vi "SpectrumViewer.vi"() -> ()   [LabVIEW 2016]
uses:
  <vilib>/Utility/miscctls.llb/LVPointDoubleTypeDef.ctl
  <vilib>/GPower/Numeric/Library/Average/AvrgDBL.vi
  <vilib>/Analysis/baseanly.llb/Mean (DBL).vi
  <vilib>/Utility/file.llb/Write Delimited Spreadsheet (DBL).vi
  <vilib>/Analysis/NI_AALBase.lvlib
  <vilib>/GPower/Numeric/GPNumeric.lvlib
panel:
  in  "Wavelength maximum":i32(slide)=374 min=374 max=761 step=1 scale=374.0..761.0
  in  "File Path":path
  in  "Save":bool
  out "Spectrum at cursor":i16[](graph)
  in  "Wavelength minimum":i32(slide)=374 min=374 max=761 step=1 scale=374.0..761.0
  in  "Intensity Graph":sgl[][](graph)
  in  "Quit":bool
  out "error out":errorcluster
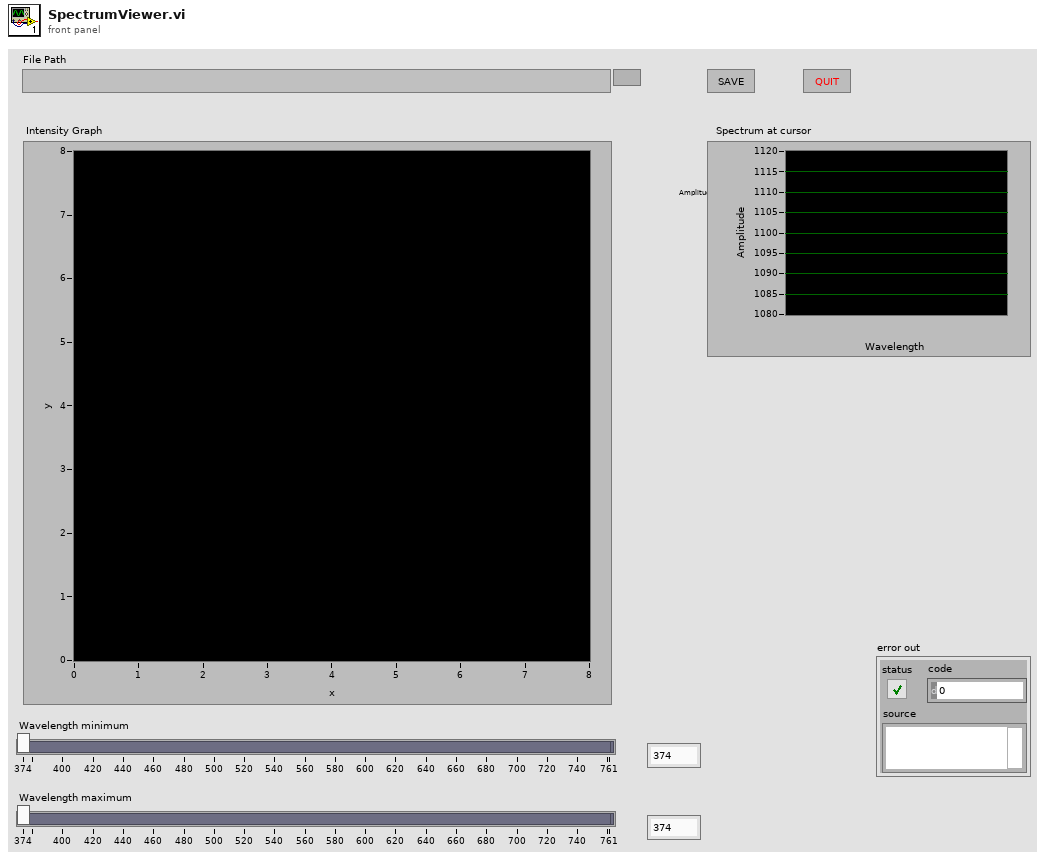
[diagram p1: front panel]
types:
  T1 = typedef "LVPointDoubleTypeDef.ctl" = cluster{"X":dbl, "Y":dbl}
  T2 = typedef "Image Type" = u32
  T3 = typedef "IMAQ Image.ctl" = refnum<image>
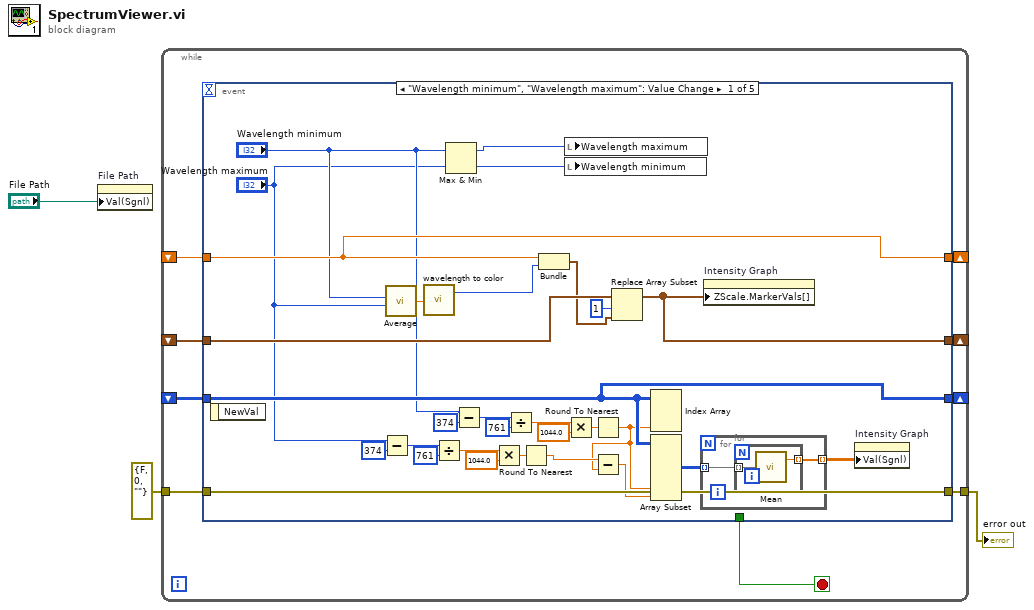
[diagram p0: block diagram]
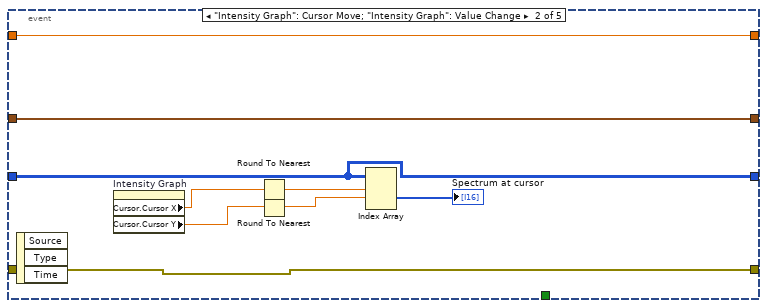
[diagram p2: hidden frame]
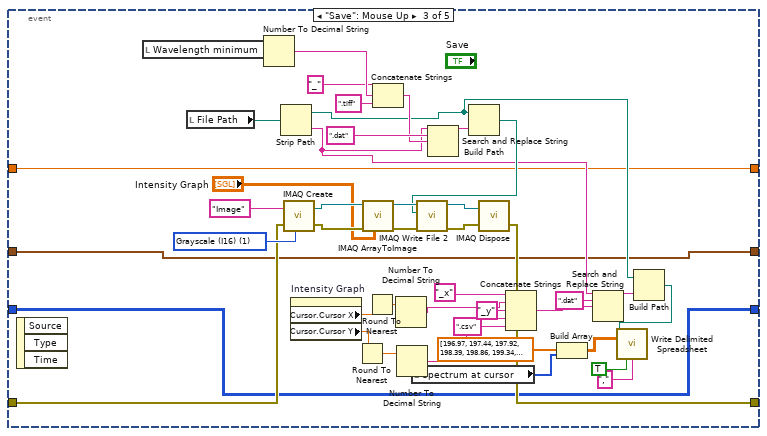
[diagram p3: hidden frame]
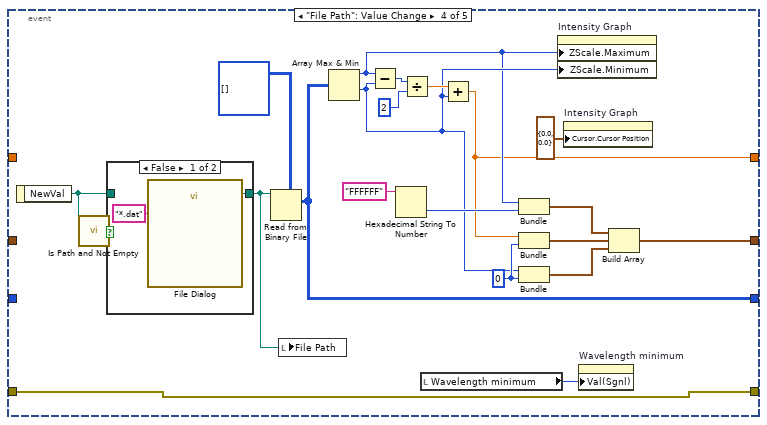
[diagram p4: hidden frame]
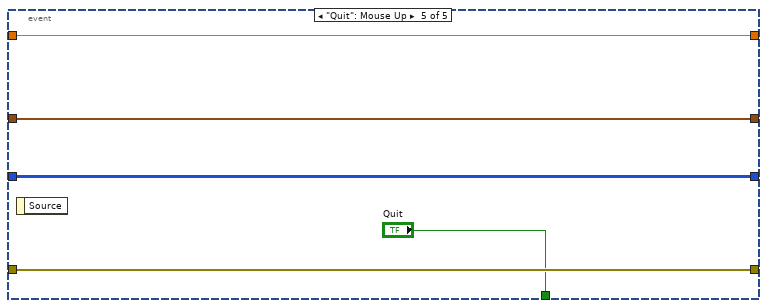
[diagram p6: hidden frame]
diagram:
  n1 = property on="File Path" class="Path"("Val(Sgnl)"="File Path") -> ()  [unwired: 2 in, 2 out]
  n2 = while {
    tunnel: errorcluster {"status"=FALSE, "code"=0, "source"=""} ("error out") -> [w11]
    tunnel: [w10] -> w3
    shift-right: [w6] -> _
    shift-left: _ -> [w12]
    shift-right: [w5] -> _
    shift-left: _ -> [w8]
    shift-right: [w4] -> _
    shift-left: _ -> [w7]
    stop <- w9 stop-if-true
    n3 = event shown="[0] \"Wavelength minimum\", \"Wavelength maximum\": Value Change" {
      selector: _ -> [_ _ _ _ _]
      dyn-events: _ -> [_ _ _ _ _]
      timeout: _ -> [_ _ _ _ _]
      tunnel: w12 -> [w23 w51 w64 _ w126]
      tunnel: w11 -> [w42 w52 w89 w112 w127]
      tunnel: [w42 w52 w90 w112 w127] -> w10
      tunnel: [_ _ _ _ "Quit"] -> w9
      tunnel: w8 -> [w41 w50 w58 _ w125]
      tunnel: w7 -> [w30 w49 w57 _ w124]
      tunnel: [w23 w51 w64 w116 w126] -> w6
      tunnel: [w31 w50 w58 w108 w125] -> w5
      tunnel: [w30 w49 w57 w99 w124] -> w4
      event "Wavelength minimum", "Wavelength maximum": Value Change {
        n4 = event-data() -> ()  [unwired: 1 in, 1 out]
        n5 = Subtract(x="Wavelength maximum", y=374) -> (x-y=w28:i32)
        n6 = call-poly <vilib>:"Average.vi"("b"="Wavelength maximum", "a"="Wavelength minimum") -> ("Average of a and b"=w17:dbl)  [unwired: 4 in]
        n7 = call "wavelength to color.vi"("Wavelength (380 - 780)"=w17) -> ("Color"=w33:u32)  [unwired: 1 out]
        n8 = Divide(x=w28, y=761) -> (x/y=w26:dbl)
        n9 = Max & Min(x="Wavelength minimum", y="Wavelength maximum") -> (max(x,y)=w13:i32, min(x,y)=w14:i32)
        n10 = Subtract(x="Wavelength minimum", y=374) -> (x-y=w38:i32)
        n11 = Multiply(x=w26, y=1044.0) -> (x*y=w24:dbl)
        n12 = Divide(x=w38, y=761) -> (x/y=w36:dbl)
        n13 = Round To Nearest(number=w24) -> (nearest integer value=w22:dbl)
        n14 = Bundle(w30, "Color"=w33) -> (w32:cluster{dbl, "Color":u32})  [unwired: 1 in]
        n15 = local write "Wavelength maximum"(w13) -> ()
        n16 = local write "Wavelength minimum"(w14) -> ()
        n17 = Multiply(x=w36, y=1044.0) -> (x*y=w34:dbl)
        n18 = Round To Nearest(number=w34) -> (nearest integer value=w21:dbl)
        n19 = Subtract(x=w22, y=w21) -> (x-y=w20:dbl)
        n20 = Replace Array Subset(array=w41, new element=w32, index=1) -> (w31:cluster{dbl, u32}[])
        n21 = Index Array(array=w23, index (dim 2)=w21) -> ()  [unwired: 2 in, 1 out]
        n22 = Array Subset(array=w23, index (dim 2)=w21, length (dim 2)=w20) -> (w19:i16[][][])  [unwired: 4 in]
        n23 = for {
          tunnel: w19 -> [w44] mode=indexing
          tunnel: [w43] -> w18 mode=indexing
          n24 = for {
            tunnel: w44 -> [w46] mode=indexing
            tunnel: [w45] -> w43 mode=indexing
            n25 = call-poly <vilib>:"Mean.vi"("X"=w46) -> ("mean"=w45:dbl)  [unwired: 1 out]
          }
        }
        n26 = property on="Intensity Graph" class="IntGraph (strict)"("ZScale.MarkerVals[]"=w31) -> ()  [unwired: 2 in, 2 out]
        n27 = property on="Intensity Graph" class="IntGraph (strict)"("Val(Sgnl)"=w18) -> ()  [unwired: 2 in, 2 out]
      }
      event "Intensity Graph": Cursor Move; "Intensity Graph": Value Change {
        n28 = event-data() -> ()  [unwired: 1 in, 3 out]
        n29 = property on="Intensity Graph" class="IntGraph (strict)"() -> ("Cursor.Cursor X"=w48:dbl, "Cursor.Cursor Y"=w47:dbl)  [unwired: 2 in, 2 out]
        n30 = Round To Nearest(number=w48) -> (nearest integer value=w55:dbl)
        n31 = Round To Nearest(number=w47) -> (nearest integer value=w54:dbl)
        n32 = Index Array(array=w51, index (dim 0)=w55, index (dim 1)=w54) -> (element=→"Spectrum at cursor":i16[])  [unwired: 1 in]
      }
      event "Save": Mouse Up {
        w91 = T2 1 items=["Grayscale (U8)", "Grayscale (I16)", "Grayscale (SGL)", "Complex (CSG)", "RGB (U32)", "HSL (U32)", "RGB (U64)", "Grayscale (U16)"] ("Image Type")
        n33 = event-data() -> ()  [unwired: 1 in, 3 out]
        n34 = local read "Wavelength minimum"() -> (w84:i32)
        n35 = local read "File Path"() -> (w80:path)
        n36 = Number To Decimal String(number=w84) -> (decimal integer string=w83:string)  [unwired: 1 in]
        n37 = Strip Path(path=w80) -> (stripped path=w78:path, name=w77:string)
        n38 = call "IMAQ Create"("Image Name"="Image", "Image Type"=w91, "error in (no error)"=w89) -> ("New Image"=w98:T3, "error out"=w96:errorcluster)  [unwired: 2 in]
        n39 = property on="Intensity Graph" class="IntGraph (strict)"() -> ("Cursor.Cursor X"=w72:dbl, "Cursor.Cursor Y"=w68:dbl)  [unwired: 2 in, 2 out]
        n40 = Round To Nearest(number=w68) -> (nearest integer value=w65:dbl)
        n41 = call "IMAQ ArrayToImage"("Image Pixels (Float)"="Intensity Graph", "error in (no error)"=w96, "Image"=w98) -> ("error out"=w95:errorcluster, "Image Out"=w94:T3)  [unwired: 7 in]
        n42 = Round To Nearest(number=w72) -> (nearest integer value=w66:dbl)
        n43 = Concatenate Strings("_" ("string"), w83, ".tiff" ("replace string (\"\")")) -> (w86:string)
        n44 = Number To Decimal String(number=w66) -> (decimal integer string=w70:string)  [unwired: 1 in]
        n45 = Number To Decimal String(number=w65) -> (decimal integer string=w67:string)  [unwired: 1 in]
        n46 = local read "Spectrum at cursor"() -> (w60:i16[])
        n47 = Search and Replace String(input string=w77, search string=".dat", replace string=w86) -> (result string=w88:string)  [unwired: 5 in, 3 out]
        n48 = Build Path(base path=w78, name or relative path=w88) -> (appended path=w81:path)
        n49 = call-poly "IMAQ Write File 2"("error in (no error)"=w95, "File Path"=w81, "Image"=w94) -> ("error out"=w92:errorcluster, "Image Out (duplicate)"=w93:T3)  [unwired: 7 in]
        n50 = call "IMAQ Dispose"("Image"=w93, "error in (no error)"=w92) -> ("error out"=w90:errorcluster)  [unwired: 4 in]
        n51 = Concatenate Strings("_x" ("string"), w70, "_y" ("string"), w67, ".csv" ("string")) -> (w75:string)
        n52 = Build Array(dbl[] [196.97, 197.44, 197.92, 198.39, 198.86, 199.34, 199.81, 200.28, 200.75, 201.22, 201.7, 202.17, 202.64, 203.11, 203.59, 204.06, 204.53, 205.0, 205.48, 205.95, 206.42, 206.89, 207.36, 207.84, 208.31, 208.78, 209.25, 209.73, 210.2, 210.67, 211.14, 211.61, 212.09, 212.56, 213.03, 213.5, 213.97, 214.44, 214.92, 215.39, 215.86, 216.33, 216.8, 217.28, 217.75, 218.22, 218.69, 219.16, 219.63, 220.11, 220.58, 221.05, 221.52, 221.99, 222.46, 222.93, 223.41, 223.88, 224.35, 224.82, 225.29, 225.76, 226.23, 226.71, 227.18, 227.65, 228.12, 228.59, 229.06, 229.53, 230.0, 230.48, 230.95, 231.42, 231.89, 232.36, 232.83, 233.3, 233.77, 234.24, 234.71, 235.19, 235.66, 236.13, 236.6, 237.07, 237.54, 238.01, 238.48, 238.95, 239.42, 239.89, 240.36, 240.84, 241.31, 241.78, 242.25, 242.72, 243.19, 243.66, 244.13, 244.6, 245.07, 245.54, 246.01, 246.48, 246.95, 247.42, 247.89, 248.36, 248.83, 249.3, 249.77, 250.24, 250.72, 251.19, 251.66, 252.13, 252.6, 253.07, 253.54, 254.01, 254.48, 254.95, 255.42, 255.89, 256.36, 256.83, 257.3, 257.77, 258.24, 258.71, 259.18, 259.65, 260.12, 260.59, 261.06, 261.53, 261.99, 262.46, 262.93, 263.4, 263.87, 264.34, 264.81, 265.28, 265.75, 266.22, 266.69, 267.16, 267.63, 268.1, 268.57, 269.04, 269.51, 269.98, 270.45, 270.92, 271.39, 271.85, 272.32, 272.79, 273.26, 273.73, 274.2, 274.67, 275.14, 275.61, 276.08, 276.55, 277.02, 277.48, 277.95, 278.42, 278.89, 279.36, 279.83, 280.3, 280.77, 281.24, 281.7, 282.17, 282.64, 283.11, 283.58, 284.05, 284.52, 284.99, 285.45, 285.92, 286.39, 286.86, 287.33, 287.8, 288.27, 288.73, 289.2, 289.67, 290.14, 290.61, 291.08, 291.54, 292.01, 292.48, 292.95, 293.42, 293.89, 294.35, 294.82, 295.29, 295.76, 296.23, 296.7, 297.16, 297.63, 298.1, 298.57, 299.04, 299.5, 299.97, 300.44, 300.91, 301.38, 301.84, 302.31, 302.78, 303.25, 303.71, 304.18, 304.65, 305.12, 305.59, 306.05, 306.52, 306.99, 307.46, 307.92, 308.39, 308.86, 309.33, 309.79, 310.26, 310.73, 311.2, 311.66, 312.13, 312.6, 313.07, 313.53, 314.0, 314.47, 314.94, 315.4, 315.87, 316.34, 316.8, 317.27, 317.74, 318.21, 318.67, 319.14, 319.61, 320.07, 320.54, 321.01, 321.48, 321.94, 322.41, 322.88, 323.34, 323.81, 324.28, 324.74, 325.21, 325.68, 326.14, 326.61, 327.08, 327.54, 328.01, 328.48, 328.94, 329.41, 329.88, 330.34, 330.81, 331.28, 331.74, 332.21, 332.68, 333.14, 333.61, 334.07, 334.54, 335.01, 335.47, 335.94, 336.41, 336.87, 337.34, 337.8, 338.27, 338.74, 339.2, 339.67, 340.14, 340.6, 341.07, 341.53, 342.0, 342.47, 342.93, 343.4, 343.86, 344.33, 344.79, 345.26, 345.73, 346.19, 346.66, 347.12, 347.59, 348.05, 348.52, 348.99, 349.45, 349.92, 350.38, 350.85, 351.31, 351.78, 352.24, 352.71, 353.18, 353.64, 354.11, 354.57, 355.04, 355.5, 355.97, 356.43, 356.9, 357.36, 357.83, 358.29, 358.76, 359.22, 359.69, 360.15, 360.62, 361.08, 361.55, 362.01, 362.48, 362.94, 363.41, 363.87, 364.34, 364.8, 365.27, 365.73, 366.2, 366.66, 367.13, 367.59, 368.06, 368.52, 368.99, 369.45, 369.92, 370.38, 370.84, 371.31, 371.77, 372.24, 372.7, 373.17, 373.63, 374.1, 374.56, 375.02, 375.49, 375.95, 376.42, 376.88, 377.35, 377.81, 378.27, 378.74, 379.2, 379.67, 380.13, 380.59, 381.06, 381.52, 381.99, 382.45, 382.91, 383.38, 383.84, 384.31, 384.77, 385.23, 385.7, 386.16, 386.63, 387.09, 387.55, 388.02, 388.48, 388.94, 389.41, 389.87, 390.33, 390.8, 391.26, 391.73, 392.19, 392.65, 393.12, 393.58, 394.04, 394.51, 394.97, 395.43, 395.9, 396.36, 396.82, 397.29, 397.75, 398.21, 398.67, 399.14, 399.6, 400.06, 400.53, 400.99, 401.45, 401.92, 402.38, 402.84, 403.31, 403.77, 404.23, 404.69, 405.16, 405.62, 406.08, 406.54, 407.01, 407.47, 407.93, 408.4, 408.86, 409.32, 409.78, 410.25, 410.71, 411.17, 411.63, 412.1, 412.56, 413.02, 413.48, 413.95, 414.41, 414.87, 415.33, 415.79, 416.26, 416.72, 417.18, 417.64, 418.11, 418.57, 419.03, 419.49, 419.95, 420.42, 420.88, 421.34, 421.8, 422.26, 422.73, 423.19, 423.65, 424.11, 424.57, 425.03, 425.5, 425.96, 426.42, 426.88, 427.34, 427.8, 428.27, 428.73, 429.19, 429.65, 430.11, 430.57, 431.04, 431.5, 431.96, 432.42, 432.88, 433.34, 433.8, 434.27, 434.73, 435.19, 435.65, 436.11, 436.57, 437.03, 437.49, 437.95, 438.42, 438.88, 439.34, 439.8, 440.26, 440.72, 441.18, 441.64, 442.1, 442.56, 443.03, 443.49, 443.95, 444.41, 444.87, 445.33, 445.79, 446.25, 446.71, 447.17, 447.63, 448.09, 448.55, 449.01, 449.47, 449.94, 450.4, 450.86, 451.32, 451.78, 452.24, 452.7, 453.16, 453.62, 454.08, 454.54, 455.0, 455.46, 455.92, 456.38, 456.84, 457.3, 457.76, 458.22, 458.68, 459.14, 459.6, 460.06, 460.52, 460.98, 461.44, 461.9, 462.36, 462.82, 463.28, 463.74, 464.2, 464.66, 465.12, 465.58, 466.04, 466.5, 466.96, 467.41, 467.87, 468.33, 468.79, 469.25, 469.71, 470.17, 470.63, 471.09, 471.55, 472.01, 472.47, 472.93, 473.39, 473.85, 474.3, 474.76, 475.22, 475.68, 476.14, 476.6, 477.06, 477.52, 477.98, 478.44, 478.89, 479.35, 479.81, 480.27, 480.73, 481.19, 481.65, 482.11, 482.57, 483.02, 483.48, 483.94, 484.4, 484.86, 485.32, 485.78, 486.23, 486.69, 487.15, 487.61, 488.07, 488.53, 488.98, 489.44, 489.9, 490.36, 490.82, 491.28, 491.73, 492.19, 492.65, 493.11, 493.57, 494.02, 494.48, 494.94, 495.4, 495.86, 496.31, 496.77, 497.23, 497.69, 498.15, 498.6, 499.06, 499.52, 499.98, 500.44, 500.89, 501.35, 501.81, 502.27, 502.72, 503.18, 503.64, 504.1, 504.55, 505.01, 505.47, 505.93, 506.38, 506.84, 507.3, 507.76, 508.21, 508.67, 509.13, 509.58, 510.04, 510.5, 510.96, 511.41, 511.87, 512.33, 512.78, 513.24, 513.7, 514.16, 514.61, 515.07, 515.53, 515.98, 516.44, 516.9, 517.35, 517.81, 518.27, 518.72, 519.18, 519.64, 520.09, 520.55, 521.01, 521.46, 521.92, 522.38, 522.83, 523.29, 523.75, 524.2, 524.66, 525.11, 525.57, 526.03, 526.48, 526.94, 527.4, 527.85, 528.31, 528.76, 529.22, 529.68, 530.13, 530.59, 531.04, 531.5, 531.96, 532.41, 532.87, 533.32, 533.78, 534.24, 534.69, 535.15, 535.6, 536.06, 536.51, 536.97, 537.43, 537.88, 538.34, 538.79, 539.25, 539.7, 540.16, 540.61, 541.07, 541.53, 541.98, 542.44, 542.89, 543.35, 543.8, 544.26, 544.71, 545.17, 545.62, 546.08, 546.53, 546.99, 547.44, 547.9, 548.35, 548.81, 549.26, 549.72, 550.17, 550.63, 551.08, 551.54, 551.99, 552.45, 552.9, 553.36, 553.81, 554.27, 554.72, 555.18, 555.63, 556.08, 556.54, 556.99, 557.45, 557.9, 558.36, 558.81, 559.27, 559.72, 560.17, 560.63, 561.08, 561.54, 561.99, 562.45, 562.9, 563.35, 563.81, 564.26, 564.72, 565.17, 565.62, 566.08, 566.53, 566.99, 567.44, 567.89, 568.35, 568.8, 569.26, 569.71, 570.16, 570.62, 571.07, 571.52, 571.98, 572.43, 572.89, 573.34, 573.79, 574.25, 574.7, 575.15, 575.61, 576.06, 576.51, 576.97, 577.42, 577.87, 578.33, 578.78, 579.23, 579.69, 580.14, 580.59, 581.05, 581.5, 581.95, 582.4, 582.86, 583.31, 583.76, 584.22, 584.67, 585.12, 585.58, 586.03, 586.48, 586.93, 587.39, 587.84, 588.29, 588.74, 589.2, 589.65, 590.1, 590.55, 591.01, 591.46, 591.91, 592.36, 592.82, 593.27, 593.72, 594.17, 594.63, 595.08, 595.53, 595.98, 596.44, 596.89, 597.34, 597.79, 598.24, 598.7, 599.15, 599.6, 600.05, 600.5, 600.96, 601.41, 601.86, 602.31, 602.76, 603.21, 603.67, 604.12, 604.57, 605.02, 605.47, 605.93, 606.38, 606.83, 607.28, 607.73, 608.18, 608.63, 609.09, 609.54, 609.99, 610.44, 610.89, 611.34, 611.79, 612.25, 612.7, 613.15, 613.6, 614.05, 614.5, 614.95, 615.4, 615.85, 616.3, 616.76, 617.21, 617.66, 618.11, 618.56, 619.01, 619.46, 619.91, 620.36, 620.81, 621.26, 621.71, 622.17, 622.62, 623.07, 623.52, 623.97, 624.42, 624.87, 625.32, 625.77, 626.22, 626.67, 627.12, 627.57, 628.02, 628.47, 628.92, 629.37, 629.82, 630.27, 630.72, 631.17, 631.62, 632.07, 632.52, 632.97, 633.42, 633.87, 634.32, 634.77, 635.22, 635.67, 636.12, 636.57, 637.02, 637.47, 637.92, 638.37, 638.82, 639.27, 639.72, 640.17, 640.62, 641.07, 641.52, 641.97, 642.42, 642.87, 643.31, 643.76, 644.21, 644.66, 645.11, 645.56, 646.01, 646.46, 646.91, 647.36, 647.81, 648.26, 648.7, 649.15, 649.6, 650.05, 650.5, 650.95, 651.4, 651.85, 652.3, 652.74, 653.19, 653.64, 654.09, 654.54, 654.99, 655.44, 655.88, 656.33, 656.78, 657.23, 657.68, 658.13, 658.58, 659.02, 659.47, 659.92, 660.37, 660.82, 661.27, 661.71, 662.16, 662.61, 663.06, 663.51, 663.95, 664.4, 664.85, 665.3, 665.75, 666.19, 666.64, 667.09, 667.54, 667.99, 668.43, 668.88, 669.33, 669.78, 670.22, 670.67, 671.12, 671.57, 672.01, 672.46, 672.91, 673.36, 673.8, 674.25, 674.7, 675.15, 675.59, 676.04, 676.49, 676.94, 677.38, 677.83, 678.28, 678.72, 679.17, 679.62, 680.07, 680.51, 680.96, 681.41, 681.85, 682.3, 682.75, 683.19, 683.64, 684.09, 684.53, 684.98, 685.43, 685.87, 686.32, 686.77, 687.21, 687.66, 688.11, 688.55, 689.0, 689.45, 689.89, 690.34, 690.79, 691.23, 691.68, 692.12, 692.57, 693.02, 693.46, 693.91, 694.36, 694.8, 695.25, 695.69, 696.14, 696.59, 697.03, 697.48, 697.92, 698.37, 698.81, 699.26, 699.71, 700.15, 700.6, 701.04, 701.49, 701.93, 702.38, 702.83, 703.27, 703.72, 704.16, 704.61, 705.05, 705.5, 705.94, 706.39, 706.83, 707.28, 707.73, 708.17, 708.62, 709.06, 709.51, 709.95, 710.4, 710.84, 711.29, 711.73, 712.18, 712.62, 713.07, 713.51, 713.96, 714.4, 714.85, 715.29, 715.74, 716.18, 716.62, 717.07, 717.51, 717.96, 718.4, 718.85, 719.29, 719.74, 720.18, 720.63, 721.07, 721.51, 721.96, 722.4, 722.85, 723.29, 723.74, 724.18, 724.62, 725.07, 725.51, 725.96, 726.4, 726.84, 727.29, 727.73, 728.18, 728.62, 729.06, 729.51, 729.95, 730.39, 730.84, 731.28, 731.73, 732.17, 732.61, 733.06, 733.5, 733.94, 734.39, 734.83, 735.27, 735.72, 736.16, 736.6, 737.05, 737.49, 737.93, 738.38, 738.82, 739.26, 739.71, 740.15, 740.59, 741.04, 741.48, 741.92, 742.37, 742.81, 743.25, 743.69, 744.14, 744.58, 745.02, 745.47, 745.91, 746.35, 746.79, 747.24, 747.68, 748.12, 748.56, 749.01, 749.45, 749.89, 750.33, 750.78, 751.22, 751.66, 752.1, 752.55, 752.99, 753.43, 753.87, 754.31, 754.76, 755.2, 755.64, 756.08, 756.52, 756.97, 757.41, 757.85, 758.29, 758.73, 759.18, 759.62, 760.06, 760.5, 760.94, 761.38, 761.83, 762.27, 762.71, 763.15, 763.59, 764.03, 764.48, 764.92, 765.36, 765.8, 766.24, 766.68, 767.12, 767.57, 768.01, 768.45, 768.89, 769.33, 769.77, 770.21, 770.65, 771.09, 771.54, 771.98, 772.42, 772.86, 773.3, 773.74, 774.18, 774.62, 775.06, 775.5, 775.94, 776.38, 776.83, 777.27, 777.71, 778.15, 778.59, 779.03, 779.47, 779.91, 780.35, 780.79, 781.23, 781.67, 782.11, 782.55, 782.99, 783.43, 783.87, 784.31, 784.75, 785.19, 785.63, 786.07, 786.51, 786.95, 787.39, 787.83, 788.27, 788.71, 789.15, 789.59, 790.03, 790.47, 790.91, 791.35, 791.79, 792.23, 792.67, 793.11, 793.55, 793.99, 794.43, 794.87, 795.3, 795.74, 796.18, 796.62, 797.06, 797.5, 797.94, 798.38, 798.82, 799.26, 799.7, 800.14, 800.57, 801.01, 801.45, 801.89, 802.33, 802.77, 803.21, 803.65, 804.09, 804.52, 804.96, 805.4, 805.84, 806.28, 806.72, 807.16, 807.59, 808.03, 808.47, 808.91, 809.35, 809.79, 810.23, 810.66, 811.1, 811.54, 811.98, 812.42, 812.85, 813.29, 813.73, 814.17, 814.61, 815.04, 815.48, 815.92, 816.36, 816.8, 817.23, 817.67, 818.11, 818.55, 818.99, 819.42, 819.86, 820.3, 820.74, 821.17, 821.61, 822.05, 822.49, 822.92, 823.36, 823.8, 824.24, 824.67, 825.11, 825.55, 825.98, 826.42, 826.86, 827.3, 827.73, 828.17, 828.61, 829.04, 829.48, 829.92, 830.35, 830.79, 831.23, 831.67, 832.1, 832.54, 832.98, 833.41, 833.85, 834.29, 834.72, 835.16, 835.59, 836.03, 836.47, 836.9, 837.34, 837.78, 838.21, 838.65, 839.09, 839.52, 839.96, 840.39, 840.83, 841.27, 841.7, 842.14, 842.58, 843.01, 843.45, 843.88, 844.32, 844.75, 845.19, 845.63, 846.06, 846.5, 846.93, 847.37, 847.8, 848.24, 848.68, 849.11, 849.55, 849.98, 850.42, 850.85, 851.29, 851.72, 852.16, 852.59, 853.03, 853.47, 853.9, 854.34, 854.77, 855.21, 855.64, 856.08, 856.51, 856.95, 857.38, 857.82, 858.25, 858.69, 859.12, 859.56, 859.99, 860.42, 860.86, 861.29, 861.73, 862.16, 862.6, 863.03, 863.47, 863.9, 864.34, 864.77, 865.2, 865.64, 866.07, 866.51, 866.94, 867.38, 867.81, 868.24, 868.68, 869.11, 869.55, 869.98, 870.42, 870.85, 871.28, 871.72, 872.15, 872.58, 873.02, 873.45, 873.89, 874.32, 874.75, 875.19, 875.62, 876.05, 876.49, 876.92, 877.35, 877.79, 878.22, 878.66, 879.09, 879.52, 879.96, 880.39, 880.82, 881.25, 881.69, 882.12, 882.55, 882.99, 883.42, 883.85, 884.29, 884.72, 885.15, 885.59, 886.02, 886.45, 886.88, 887.32, 887.75, 888.18, 888.61, 889.05, 889.48, 889.91, 890.34, 890.78, 891.21, 891.64, 892.07, 892.51, 892.94, 893.37, 893.8, 894.24, 894.67, 895.1, 895.53, 895.96, 896.4, 896.83, 897.26, 897.69, 898.12, 898.56, 898.99, 899.42, 899.85, 900.28, 900.72, 901.15, 901.58, 902.01, 902.44, 902.87, 903.31, 903.74, 904.17, 904.6, 905.03, 905.46, 905.89, 906.33, 906.76, 907.19, 907.62, 908.05, 908.48, 908.91, 909.34, 909.77, 910.21, 910.64, 911.07, 911.5, 911.93, 912.36, 912.79, 913.22, 913.65, 914.08, 914.51, 914.95, 915.38, 915.81, 916.24, 916.67, 917.1, 917.53, 917.96, 918.39, 918.82, 919.25, 919.68, 920.11, 920.54, 920.97, 921.4, 921.83, 922.26, 922.69, 923.12, 923.55, 923.98, 924.41, 924.84, 925.27, 925.7, 926.13, 926.56, 926.99, 927.42, 927.85, 928.28, 928.71, 929.14, 929.57, 930.0, 930.43, 930.86, 931.29, 931.72, 932.15, 932.57, 933.0, 933.43, 933.86, 934.29, 934.72, 935.15, 935.58, 936.01, 936.44, 936.87, 937.3, 937.72, 938.15, 938.58, 939.01, 939.44, 939.87, 940.3, 940.73, 941.15, 941.58, 942.01, 942.44, 942.87, 943.3, 943.73, 944.15, 944.58, 945.01, 945.44, 945.87, 946.3, 946.72, 947.15, 947.58, 948.01, 948.44, 948.87, 949.29, 949.72, 950.15, 950.58, 951.01, 951.43, 951.86, 952.29, 952.72, 953.14, 953.57, 954.0, 954.43, 954.85, 955.28, 955.71, 956.14, 956.56, 956.99, 957.42, 957.85, 958.27, 958.7, 959.13, 959.56, 959.98, 960.41, 960.84, 961.26, 961.69, 962.12, 962.55, 962.97, 963.4, 963.83, 964.25, 964.68, 965.11, 965.53, 965.96, 966.39, 966.81, 967.24, 967.67, 968.09, 968.52, 968.95, 969.37, 969.8, 970.23, 970.65, 971.08, 971.51, 971.93, 972.36, 972.78, 973.21, 973.64, 974.06, 974.49, 974.91, 975.34, 975.77, 976.19, 976.62, 977.04, 977.47, 977.9, 978.32, 978.75, 979.17, 979.6, 980.02, 980.45, 980.88, 981.3, 981.73, 982.15, 982.58, 983.0, 983.43, 983.85, 984.28, 984.7, 985.13, 985.55, 985.98, 986.4, 986.83, 987.25, 987.68, 988.1, 988.53, 988.95, 989.38, 989.8, 990.23, 990.65, 991.08, 991.5, 991.93, 992.35, 992.78, 993.2, 993.63, 994.05, 994.48, 994.9, 995.32, 995.75, 996.17, 996.6, 997.02, 997.45, 997.87, 998.29, 998.72, 999.14, 999.57, 999.99, 1000.41, 1000.84, 1001.26, 1001.69, 1002.11, 1002.53, 1002.96, 1003.38, 1003.81, 1004.23, 1004.65, 1005.08, 1005.5, 1005.92, 1006.35, 1006.77, 1007.19, 1007.62, 1008.04, 1008.46, 1008.89, 1009.31, 1009.73, 1010.16, 1010.58, 1011.0, 1011.43, 1011.85, 1012.27, 1012.7, 1013.12, 1013.54, 1013.96, 1014.39, 1014.81, 1015.23, 1015.66, 1016.08, 1016.5, 1016.92, 1017.35, 1017.77, 1018.19, 1018.61, 1019.04, 1019.46, 1019.88, 1020.3, 1020.73, 1021.15, 1021.57, 1021.99, 1022.41, 1022.84, 1023.26, 1023.68, 1024.1, 1024.53, 1024.95, 1025.37, 1025.79, 1026.21, 1026.63, 1027.06, 1027.48, 1027.9, 1028.32, 1028.74, 1029.17, 1029.59, 1030.01, 1030.43, 1030.85, 1031.27, 1031.69, 1032.12, 1032.54, 1032.96, 1033.38, 1033.8, 1034.22, 1034.64, 1035.06, 1035.49, 1035.91, 1036.33, 1036.75, 1037.17, 1037.59, 1038.01, 1038.43, 1038.85, 1039.27, 1039.7, 1040.12, 1040.54, 1040.96, 1041.38, 1041.8, 1042.22, 1042.64, 1043.06, 1043.48, 1043.9, 1044.32, 1044.74, 1045.16, 1045.58, 1046.0, 1046.42, 1046.84, 1047.26, 1047.68, 1048.1, 1048.52, 1048.94, 1049.36, 1049.78, 1050.2, 1050.62, 1051.04, 1051.46, 1051.88, 1052.3, 1052.72, 1053.14, 1053.56, 1053.98, 1054.4, 1054.82, 1055.24, 1055.66, 1056.08, 1056.5, 1056.92, 1057.34, 1057.76, 1058.17, 1058.59, 1059.01, 1059.43, 1059.85, 1060.27, 1060.69, 1061.11, 1061.53, 1061.95, 1062.36, 1062.78, 1063.2, 1063.62, 1064.04, 1064.46, 1064.88, 1065.3, 1065.71, 1066.13, 1066.55, 1066.97, 1067.39, 1067.81, 1068.23, 1068.64, 1069.06, 1069.48, 1069.9, 1070.32, 1070.74, 1071.15, 1071.57, 1071.99, 1072.41, 1072.83, 1073.24, 1073.66, 1074.08, 1074.5, 1074.91, 1075.33, 1075.75, 1076.17, 1076.59, 1077.0, 1077.42, 1077.84, 1078.26, 1078.67, 1079.09, 1079.51, 1079.93, 1080.34, 1080.76, 1081.18, 1081.59, 1082.01, 1082.43, 1082.85, 1083.26, 1083.68, 1084.1, 1084.51, 1084.93, 1085.35, 1085.77, 1086.18, 1086.6, 1087.02, 1087.43, 1087.85, 1088.27, 1088.68, 1089.1, 1089.52, 1089.93, 1090.35, 1090.77, 1091.18, 1091.6, 1092.01, 1092.43, 1092.85, 1093.26, 1093.68, 1094.1, 1094.51, 1094.93, 1095.34, 1095.76, 1096.18, 1096.59, 1097.01, 1097.42, 1097.84, 1098.26, 1098.67, 1099.09, 1099.5, 1099.92, 1100.33, 1100.75, 1101.16, 1101.58, 1102.0, 1102.41, 1102.83, 1103.24, 1103.66, 1104.07, 1104.49, 1104.9, 1105.32, 1105.73, 1106.15, 1106.56, 1106.98, 1107.39, 1107.81, 1108.22, 1108.64, 1109.05, 1109.47, 1109.88, 1110.3, 1110.71, 1111.13, 1111.54, 1111.96, 1112.37, 1112.79, 1113.2, 1113.61, 1114.03, 1114.44, 1114.86, 1115.27, 1115.69, 1116.1, 1116.52, 1116.93, 1117.34, 1117.76, 1118.17, 1118.59, 1119.0, 0.0] ("all rows"), w60) -> (w59:dbl[][])
        n53 = Search and Replace String(input string=w77, search string=".dat", replace string=w75) -> (result string=w79:string)  [unwired: 5 in, 3 out]
        n54 = Build Path(base path=w78, name or relative path=w79) -> (appended path=w73:path)
        n55 = call-poly <vilib>:"Write Delimited Spreadsheet.vi"("file path (dialog if empty)"=w73, "2D data"=w59, "transpose? (no:F)"=TRUE ("transpose? (F)"), "delimiter (\\t)"="," ("delimiter (\\t)")) -> ()  [unwired: 10 in, 2 out]
      }
      event "File Path": Value Change {
        w107 = u32 0
        n56 = event-data() -> ("NewVal"=w101:path)  [unwired: 1 in]
        n57 = call <vilib>:"Is Path and Not Empty.vi"("path"=w101) -> ("Is Path and Not Empty?"=w102:bool)  [unwired: 4 in]
        n58 = case shown="False" w102 {
          tunnel: [w121 w122] -> w100
          tunnel: w101 -> [_ w122]
          frame False {
            n59 = call "File Dialog"("pattern (all files)"="*.dat") -> ("selected path"=w121:path)  [unwired: 11 in, 3 out]
          }
          frame True {
          }
        }
        n60 = Read from Binary File(5:i16[][][] [], 11:w100) -> (2:w116:i16[][][])  [unwired: 4 in, 3 out]
        n61 = local write "File Path"(w100) -> ()
        n62 = Array Max & Min(array=w116) -> (max value=w103:i16, min value=w104:i16)  [unwired: 2 out]
        n63 = Subtract(x=w103, y=w104) -> (x-y=w115:i16)
        n64 = Hexadecimal String To Number(string="FFFFFF") -> (number=w105:u32)  [unwired: 2 in, 1 out]
        n65 = Divide(x=w115, y=i16 2) -> (x/y=w113:dbl)
        n66 = local read "Wavelength minimum"() -> (w118:i32)
        n67 = Add(x=w113, y=w104) -> (x+y=w99:dbl)
        n68 = Bundle(w103, w105) -> (w111:cluster{i16, u32})  [unwired: 1 in]
        n69 = Bundle(w99, w107) -> (w110:cluster{dbl, u32})  [unwired: 1 in]
        n70 = Bundle(w104, w107) -> (w109:cluster{i16, u32})  [unwired: 1 in]
        n71 = property on="Intensity Graph" class="IntGraph (strict)"("ZScale.Maximum"=w103, "ZScale.Minimum"=w104) -> ()  [unwired: 2 in, 2 out]
        n72 = property on="Intensity Graph" class="IntGraph (strict)"("Cursor.Cursor Position"=T1 {"X"=0.0, "Y"=0.0}) -> ()  [unwired: 2 in, 2 out]
        n73 = property on="Wavelength minimum" class="Slide (strict)"("Val(Sgnl)"=w118) -> ()  [unwired: 2 in, 2 out]
        n74 = Build Array(w111, w110, w109) -> (w108:cluster{dbl, u32}[])
      }
      event "Quit": Mouse Up {
        n75 = event-data() -> ()  [unwired: 1 in, 1 out]
      }
    }
  }
  "error out" <- w3
